vi "Open.vi"(6 "error in (no error)":errorcluster, 9 "Device Index":u32) -> (0 "error out":errorcluster, 3 "DeviceRefnum Out":u64)   [LabVIEW 2014]
doc: "RTLSDR_API int rtlsdr_open(rtlsdr_dev_t **dev, uint32_t index);"
panel:
  in  "DeviceRefnum":u64
  out "function return":i32
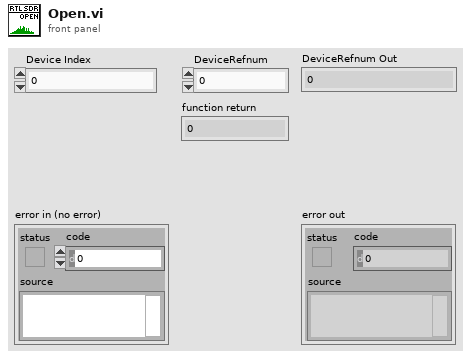
[diagram p1: front panel]
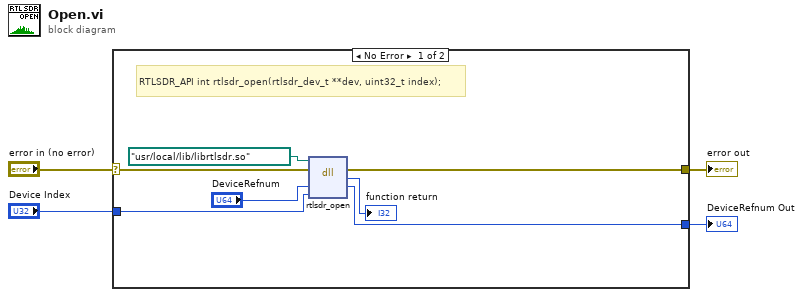
[diagram p0: block diagram]
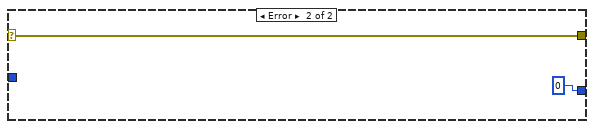
[diagram p2: hidden frame]
diagram:
  n1 = case shown="No Error" "error in (no error)" {
    selector: "error in (no error)" -> [w6 w13]
    tunnel: "Device Index" -> [w10 _]
    tunnel: [w9 w13] -> w3
    tunnel: [w8 u64 0 ("DeviceRefnum")] -> w2
    frame No Error {
      # "RTLSDR_API int rtlsdr_open(rtlsdr_dev_t **dev, uint32_t index);"
      n2 = dll-call lib="C:/Program Files (x86)/National Instruments/LabVIEW 2016/user.lib/rtlsdr/rtlsdr.*" fn="rtlsdr_open"(path in=path "/usr/local/lib/librtlsdr.so", error in=w6, "DeviceRefnum"="DeviceRefnum", "index"=w10) -> (error out=w9:errorcluster, "return type"=→"function return":i32, "DeviceRefnum"=w8:u64)  [unwired: 2 in, 1 out]
    }
    frame Error {
    }
  }
  "error out" <- w3
  "DeviceRefnum Out" <- w2
